vi "Start AC Source.vi"(8 "error in (no error)":errorcluster, 10 "Signal frequency  (Hz)":dbl, 11 "AC source":T1={"AC Source type"=enum."Agilent 331xxA to 332xxA", "awg lib session"={"type"=enum."Agilent 331xxA to 332xxA", "VISA"="", "enable 10MHz ref"=FALSE, "cmi ckd2"={"VISA"="", "clock source"=enum."Auto", "manual ref clk"=FALSE, "ref clock [Hz]"=0.0, "div mode"=enum."Set divisor directly"}, "cmi sync v3"={"VISA"="", "baud rate [bd/s]"=115200, "source"=enum."Auto", "hv range"=enum."1kV", "fsrc is fixed"=FALSE, "fsrc [Hz]"=10000000.0, "freq integ [s]"=1.0, "freq filter"=5, "trig level"=enum."TTL 5V", "chn1 mode"=enum."Source divider", "chn1 level"=enum."Positive 5V", "chn2 mode"=enum."Source divider", "chn2 level"=enum."Positive 5V", "chn2 div"=1, "chn3 mode"=enum."Chn 1 Active", "chn3 level"=enum."Positive 5V", "chn1 div entry"=enum."Calculate nearest divisor from measured fx", "chn1 dev limit [%]"=1.0, "chn1 check dev"=FALSE}, "trigger"={"source"=enum."Immediate", "level [V]"=0.0, "coupling"=enum."DC", "slope"=enum."POS"}, "HMF2500 cfg"={"Baud Rate"=9600, "Parity"=0, "Data Bits"=8, "Flow Control"=4}}, "DAQmx Device Name"="PXI2Slot6"} {"awg lib session"."HMF2500 cfg"."Flow Control" items=["None", "XON/XOFF", "RTS/CTS", "XON/XOFF & RTS/CTS", "DTR/DSR", "XON/XOFF & DTR/DSR"]; "awg lib session"."HMF2500 cfg"."Data Bits" items=["7"=7, "8"=8]; "awg lib session"."HMF2500 cfg"."Parity" items=["None", "Odd", "Even", "Mark", "Space"]; "awg lib session"."HMF2500 cfg"."Baud Rate" items=["300"=300, "600"=600, "1200"=1200, "2400"=2400, "4800"=4800, "9600"=9600, "19200"=19200]; "awg lib session"."cmi sync v3"."chn2 div" min=1 max=100000000 step=1; "awg lib session"."cmi sync v3"."fsrc [Hz]" format="%_8p"}) -> (0 "error out":errorcluster, 3 "AC source out":T1={"AC Source type"=enum."Agilent 331xxA to 332xxA", "awg lib session"={"type"=enum."Agilent 331xxA to 332xxA", "VISA"="", "enable 10MHz ref"=FALSE, "cmi ckd2"={"VISA"="", "clock source"=enum."Auto", "manual ref clk"=FALSE, "ref clock [Hz]"=0.0, "div mode"=enum."Set divisor directly"}, "cmi sync v3"={"VISA"="", "baud rate [bd/s]"=115200, "source"=enum."Auto", "hv range"=enum."1kV", "fsrc is fixed"=FALSE, "fsrc [Hz]"=10000000.0, "freq integ [s]"=1.0, "freq filter"=5, "trig level"=enum."TTL 5V", "chn1 mode"=enum."Source divider", "chn1 level"=enum."Positive 5V", "chn2 mode"=enum."Source divider", "chn2 level"=enum."Positive 5V", "chn2 div"=1, "chn3 mode"=enum."Chn 1 Active", "chn3 level"=enum."Positive 5V", "chn1 div entry"=enum."Calculate nearest divisor from measured fx", "chn1 dev limit [%]"=1.0, "chn1 check dev"=FALSE}, "trigger"={"source"=enum."Immediate", "level [V]"=0.0, "coupling"=enum."DC", "slope"=enum."POS"}, "HMF2500 cfg"={"Baud Rate"=9600, "Parity"=0, "Data Bits"=8, "Flow Control"=4}}, "DAQmx Device Name"="PXI2Slot6"} {"awg lib session"."HMF2500 cfg"."Flow Control" items=["None", "XON/XOFF", "RTS/CTS", "XON/XOFF & RTS/CTS", "DTR/DSR", "XON/XOFF & DTR/DSR"]; "awg lib session"."HMF2500 cfg"."Data Bits" items=["7"=7, "8"=8]; "awg lib session"."HMF2500 cfg"."Parity" items=["None", "Odd", "Even", "Mark", "Space"]; "awg lib session"."HMF2500 cfg"."Baud Rate" items=["300"=300, "600"=600, "1200"=1200, "2400"=2400, "4800"=4800, "9600"=9600, "19200"=19200]; "awg lib session"."cmi sync v3"."chn2 div" min=1 max=100000000 step=1; "awg lib session"."cmi sync v3"."fsrc [Hz]" format="%_8p"})   [LabVIEW 2020]
uses:
  Type definitions/AC Source.ctl
  Type definitions/AC Source type.ctl
  external libraries/AWG/AWG Session.ctl
  external libraries/AWG/AWG Type.ctl
  external libraries/AWG/CMI Clock Divider v2/CMI ckd2 Session.ctl
  external libraries/AWG/CMI Clock Divider v2/CMI ckd2 Source Mode.ctl
  external libraries/AWG/CMI Clock Divider v2/CMI ckd2 Divisor Mode.ctl
  external libraries/AWG/CMI Sync V3/CMI Sync V3 session.ctl
  external libraries/AWG/CMI Sync V3/Configure/CMI Sync V3 Reference Clock Source.ctl
  external libraries/AWG/CMI Sync V3/Configure/CMI Sync V3 HV input Range.ctl
  external libraries/AWG/CMI Sync V3/Configure/CMI Sync V3 Trigger Input Level.ctl
  external libraries/AWG/CMI Sync V3/Configure/CMI Sync V3 Channel 1 Mode.ctl
  external libraries/AWG/CMI Sync V3/Configure/CMI Sync V3 Channel Output Levels.ctl
  external libraries/AWG/CMI Sync V3/Configure/CMI Sync V3 Channel 2 Mode.ctl
  external libraries/AWG/CMI Sync V3/Configure/CMI Sync V3 Channel 3 Mode.ctl
  external libraries/AWG/CMI Sync V3/Configure/CMI Sync V3 Channel 1 Divisor Entry Mode.ctl
  external libraries/externals needed for AWG/ADC Trig Config.ctl
  external libraries/externals needed for AWG/ADC Trig Mode Source.ctl
  external libraries/externals needed for AWG/ADC Trig Coupling.ctl
  external libraries/externals needed for AWG/ADC Trig Slope.ctl
  external libraries/AWG/RaS HMF2500/HMF2500 Config.ctl
  external libraries/AWG/AWG.lvlib
  external libraries/AWG/AWG Clock Setup Mode.ctl
  external libraries/externals needed for AWG/3458A Sampling Rate.ctl
  external libraries/Fluke 5XXX Series Multicalibrator/Fluke 5XXX Series Multicalibrators.lvlib
  external libraries/AWG/CMI Sync V3/CMI Sync Unit V3.lvlib
panel:
  in  "Signal amplitude (V)":dbl
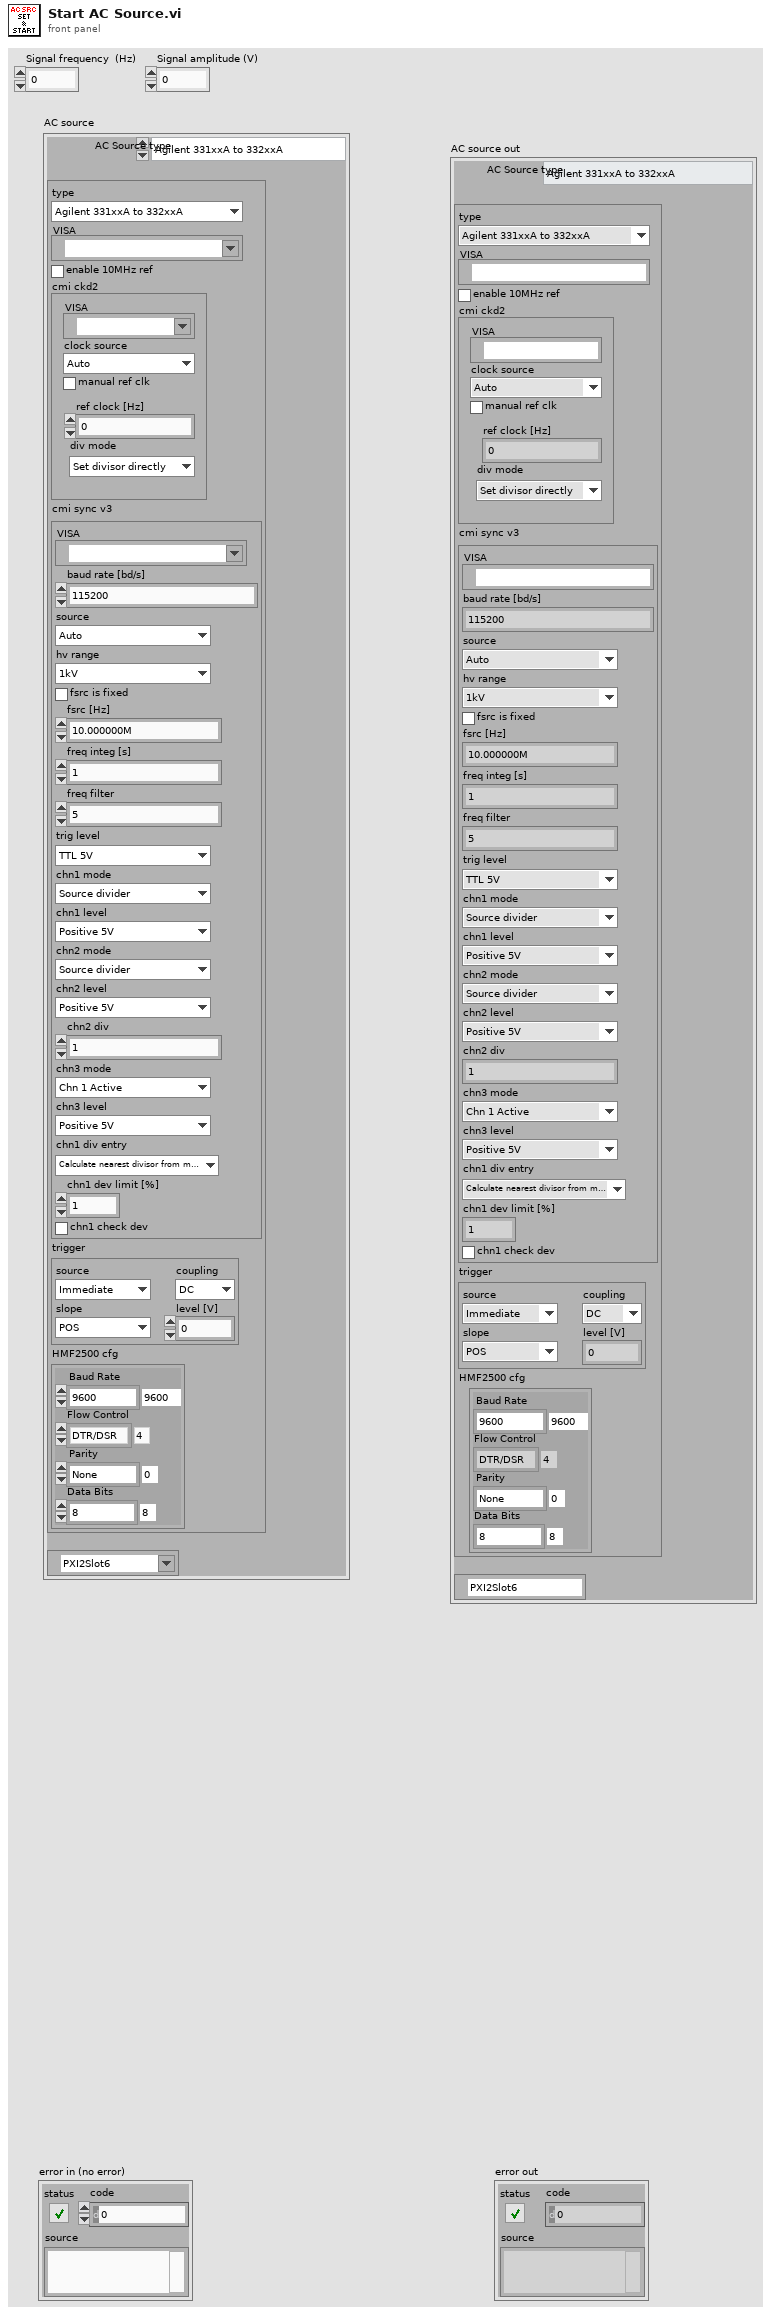
[diagram p1: front panel]
types:
  T1 = typedef "AC Source.ctl" = cluster{"AC Source type":T2, "awg lib session":T3, "DAQmx Device Name":tag}
  T2 = typedef "AC Source type.ctl" = enum16{"Agilent 331xxA to 332xxA", "Agilent 335xxA to 336xxA", "Tektronix AFG3101C", "R&S HMF25xx", "CMI Clock Divider v2", "CMI Sync Unit V3", "NI DAQ", "Fluke 5XXX calibrator", "dummy"}
  T3 = typedef "AWG.lvlib/AWG Session.ctl" = cluster{"type":T4, "VISA":refnum<visa-resource-name>, "enable 10MHz ref":bool, "cmi ckd2":T5, "cmi sync v3":T8, "trigger":T17, "HMF2500 cfg":T21}
  T4 = typedef "AWG.lvlib/AWG Type.ctl" = enum16{"Agilent 331xxA to 332xxA", "Agilent 335xxA to 336xxA", "Tektronix AFG3101C", "R&S HMF25xx", "CMI Clock Divider v2", "CMI Sync Unit V3", "dummy"}
  T5 = typedef "AWG.lvlib/CMI ckd2 Session.ctl" = cluster{"VISA":refnum<visa-resource-name>, "clock source":T6, "manual ref clk":bool, "ref clock [Hz]":dbl, "div mode":T7}
  T6 = typedef "AWG.lvlib/CMI ckd2 Source Mode.ctl" = enum16{"Auto", "LF clock", "HF clock", "Internal"}
  T7 = typedef "AWG.lvlib/CMI ckd2 Divisor Mode.ctl" = enum16{"Set divisor directly", "Set divisor by frequency"}
  T8 = typedef "AWG.lvlib/CMI Sync Unit V3.lvlib/CMI Sync V3 session.ctl" = cluster{"VISA":refnum<visa-resource-name>, "baud rate [bd/s]":i32, "source":T9, "hv range":T10, "fsrc is fixed":bool, "fsrc [Hz]":dbl, "freq integ [s]":dbl, "freq filter":i32, "trig level":T11, "chn1 mode":T12, "chn1 level":T13, "chn2 mode":T14, "chn2 level":T13, "chn2 div":i32, "chn3 mode":T15, "chn3 level":T13, "chn1 div entry":T16, "chn1 dev limit [%]":dbl, "chn1 check dev":bool}
  T9 = typedef "AWG.lvlib/CMI Sync Unit V3.lvlib/CMI Sync V3 Reference Clock Source.ctl" = enum16{"Auto", "Internal", "Logic", "Sine", "HV"}
  T10 = typedef "AWG.lvlib/CMI Sync Unit V3.lvlib/CMI Sync V3 HV input Range.ctl" = enum16{"10V", "60V", "250V", "1kV"}
  T11 = typedef "AWG.lvlib/CMI Sync Unit V3.lvlib/CMI Sync V3 Trigger Input Level.ctl" = enum16{"LVCMOS 3V3", "TTL 5V"}
  T12 = typedef "AWG.lvlib/CMI Sync Unit V3.lvlib/CMI Sync V3 Channel 1 Mode.ctl" = enum16{"Source divider", "DDS absolute", "DDS ratio", "DDS ratio M/N"}
  T13 = typedef "AWG.lvlib/CMI Sync Unit V3.lvlib/CMI Sync V3 Channel Output Levels.ctl" = enum16{"Positive 3V3", "Negative 3V3", "Positive 5V", "Negative 5V"}
  T14 = typedef "AWG.lvlib/CMI Sync Unit V3.lvlib/CMI Sync V3 Channel 2 Mode.ctl" = enum16{"Source divider", "Chn 1 divide"}
  T15 = typedef "AWG.lvlib/CMI Sync Unit V3.lvlib/CMI Sync V3 Channel 3 Mode.ctl" = enum16{"Chn 1 Active", "Chn 2 Active", "Chn 1 Trigger", "Chn 2 Trigger", "Gate", "PPS", "10MHz"}
  T16 = typedef "AWG.lvlib/CMI Sync Unit V3.lvlib/CMI Sync V3 Channel 1 Divisor Entry Mode.ctl" = enum16{"Set divisor directly", "Calculate nearest divisor from measured fx"}
  T17 = typedef "ADC Trig Config.ctl" = cluster{"source":T18, "level [V]":dbl, "coupling":T19, "slope":T20}
  T18 = typedef "ADC Trig Mode Source.ctl" = enum16{"Immediate", "External", "Level"}
  T19 = typedef "ADC Trig Coupling.ctl" = enum16{"DC", "AC"}
  T20 = typedef "ADC Trig Slope.ctl" = enum16{"POS", "NEG"}
  T21 = typedef "AWG.lvlib/HMF2500 Config.ctl" = cluster{"Baud Rate":u32, "Parity":u16, "Data Bits":u16, "Flow Control":u16}
  T22 = typedef "3458A Sampling Rate.ctl" = cluster{"freq mode":T23, "fs [Hz]":dbl, "fref [Hz]":dbl, "mul":dbl, "div":dbl, "Amplitude (V)":dbl}
  T23 = typedef "AWG.lvlib/AWG Clock Setup Mode.ctl" = enum16{"fs or Ts", "fs or Ts with fref", "fref/N", "fref*M/N", "fref*Ratio"}
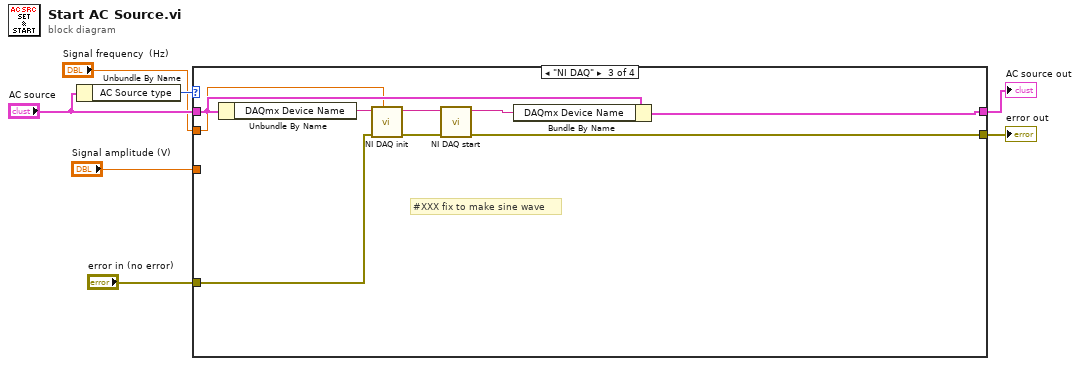
[diagram p0: block diagram]
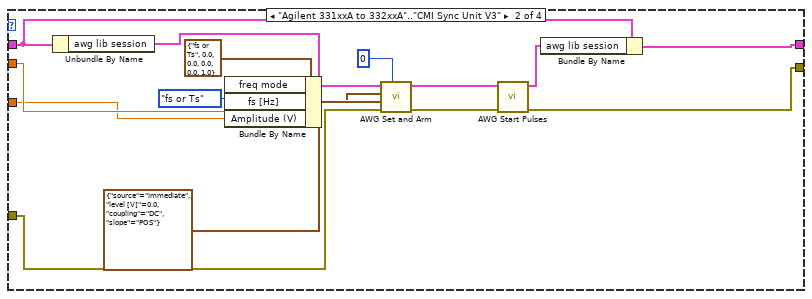
[diagram p3: hidden frame]
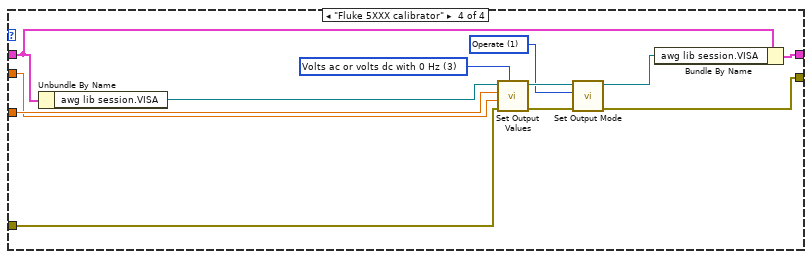
[diagram p4: hidden frame]
diagram:
  n1 = Unbundle By Name("AC source") -> ("AC Source type"=w5:T2)
  n2 = case shown="\"NI DAQ\"" w5 {
    tunnel: "error in (no error)" -> [w9 w14 w27 w45]
    tunnel: [w9 w24 w33 w37] -> w6
    tunnel: "AC source" -> [w8 w21 w32 w44]
    tunnel: [w8 w22 w31 w43] -> w3
    tunnel: "Signal frequency  (Hz)" -> [_ w13 w25 w39]
    tunnel: "Signal amplitude (V)" -> [_ w10 _ w40]
    frame "dummy" {
    }
    frame "Agilent 331xxA to 332xxA".."CMI Sync Unit V3" {
      n3 = Unbundle By Name(w21) -> ("awg lib session"=w15:T3)
      n4 = Bundle By Name(cluster=T22 {"freq mode"=enum."fs or Ts", "fs [Hz]"=0.0, "fref [Hz]"=0.0, "mul"=0.0, "div"=0.0, "Amplitude (V)"=1.0} ("sampling rate"), "freq mode"=AWG_Clock_Setup_Mode."fs or Ts", "fs [Hz]"=w13, "Amplitude (V)"=w10) -> (w18:T22)
      n5 = call "AWG Set and Arm.vi"("pulse count (0: infinite)"=0, "error in (no error)"=w14, "trigger"=T17 {"source"=enum."Immediate", "level [V]"=0.0, "coupling"=enum."DC", "slope"=enum."POS"}, "sampling rate"=w18, "awg session in"=w15) -> ("error out"=w17:errorcluster, "awg session out"=w16:T3)  [unwired: 5 in]
      n6 = call "AWG Start Pulses.vi"("error in (no error)"=w17, "awg session in"=w16) -> ("error out"=w24:errorcluster, "awg session out"=w23:T3)  [unwired: 8 in]
      n7 = Bundle By Name(cluster=w21, "awg lib session"=w23) -> (w22:T1)
    }
    frame "NI DAQ" {
      # "#XXX fix to make sine wave"
      n8 = Unbundle By Name(w32) -> ("DAQmx Device Name"=w26:tag)
      n9 = call "NI DAQ init.vi"("trigger frequency"=w25, "error in"=w27, "DAQmx Device Name"=w26) -> ("error out"=w29:errorcluster, "DAQmx Device Name Out"=w28:tag)  [unwired: 7 in]
      n10 = call "NI DAQ start.vi"("error in"=w29, "DAQmx Device Name"=w28) -> ("error out"=w33:errorcluster, "DAQmx Device Name Out"=w30:tag)  [unwired: 8 in]
      n11 = Bundle By Name(cluster=w32, "DAQmx Device Name"=w30) -> (w31:T1)
    }
    frame "Fluke 5XXX calibrator" {
      w34 = u32 1 items=["Standby", "Operate"] ("Output Mode (0: Standby)")
      w41 = u32 3 items=["Amplitude", "Volts dc or update volts ac", "Volts ac dBm update", "Volts ac or volts dc with 0 Hz", "Volts ac in dBm", "Current dc or update current ac", "Current ac", "Update frequency", "Resistance", "Capacitance", "Temperature (Celsius)", "Temperature (Fahrenheit)", "Power dc or update power ac", "Power ac", "Dual volts dc or update dual ac", "Dual volts ac in volts", "Power ac in dBm update", "Power ac in dBm", "Dual volts ac in dBm update", "Dual volts ac in dBm"] ("Output Value(s) (0 - Amplitude)")
      n12 = Unbundle By Name(w44) -> ("awg lib session.VISA"=w42:refnum<visa-resource-name>)
      n13 = call "Set Output Values.vi"("Output Value(s) (0 - Amplitude)"=w41, "error in (no error)"=w45, "Secondary Value (0.0)"=w39, "Primary Value (0.0)"=w40, "VISA resource name"=w42) -> ("error out"=w38:errorcluster, "VISA resource name out"=w36:refnum<visa-resource-name>)  [unwired: 5 in]
      n14 = call "Set Output Mode.vi"("error in (no error)"=w38, "Output Mode (0: Standby)"=w34, "VISA resource name"=w36) -> ("error out"=w37:errorcluster, "VISA resource name out"=w35:refnum<visa-resource-name>)  [unwired: 7 in]
      n15 = Bundle By Name(cluster=w44, "awg lib session.VISA"=w35) -> (w43:T1)
    }
  }
  "error out" <- w6
  "AC source out" <- w3
